vi "Insert Panel at Index.vi"(8 "error in (no error)":errorcluster, 9 "2D Index":T1, 10 "ArrayPanel":refnum<class "ArrayPanel.lvclass">, 11 "2DArrayManager in":refnum<class "2DArrayManager.lvclass">) -> (0 "error out":errorcluster, 1 "Element Replaced":bool, 2 "Replaced Element":refnum<class "ArrayPanel.lvclass">, 3 "2DArrayManager out":refnum<class "2DArrayManager.lvclass">)   [LabVIEW 2020, in "OOPanel.lvlib" / "2DArrayManager.lvclass"]
uses:
  2DArrayManager.lvclass
  ArrayPanel/ArrayPanel.lvclass
  2D Index.ctl
  2DArrayManager.lvclass/2DArrayManager.ctl
  ArrayPanel/ArrayPanel.lvclass/ArrayPanel.ctl
  ec524e60-b0c9-4dc9-b7a4-63c787fc97ef.vi
  <vilib>/Comparison/Equal/Equal Functor/Equal Functor.lvclass
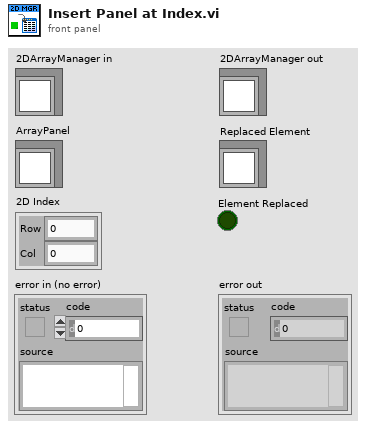
[diagram p1: front panel]
types:
  T1 = typedef "OOPanel.lvlib/2DArrayManager.lvclass/2D Index.ctl" = cluster{"Row":i32, "Col":i32}
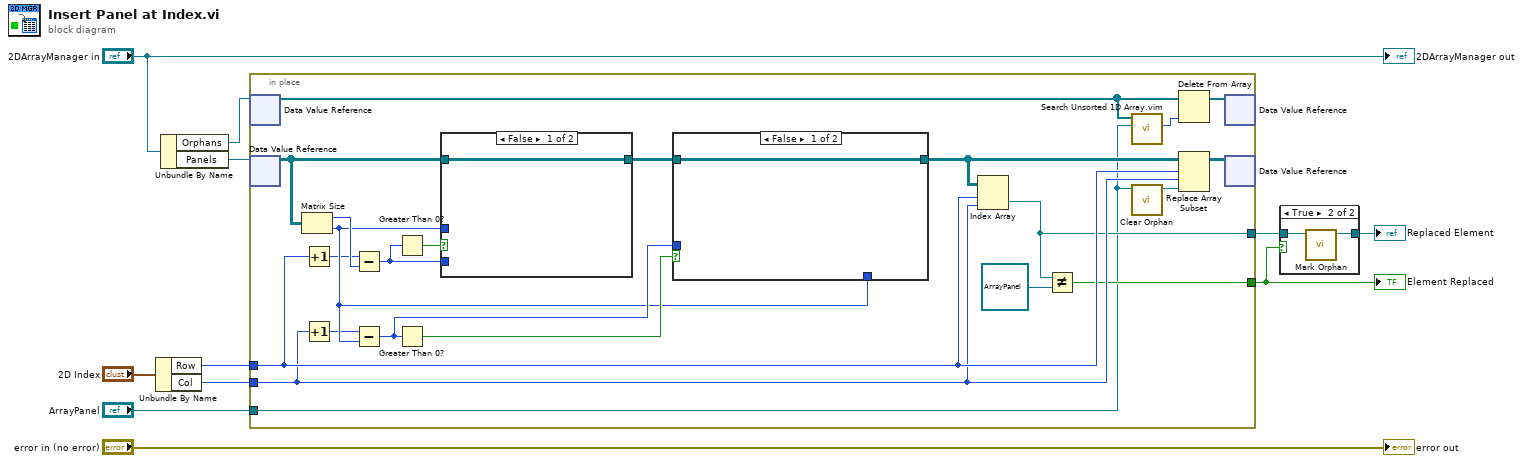
[diagram p0: block diagram]
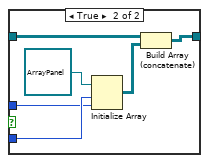
[diagram p2: hidden frame]
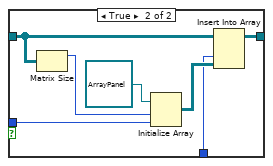
[diagram p3: hidden frame]
diagram:
  n1 = Unbundle By Name("2D Index") -> ("Row"=w7:i32, "Col"=w6:i32)
  n2 = Unbundle By Name("2DArrayManager in") -> ("Orphans"=w1:refnum<data-value>, "Panels"=w9:refnum<data-value>)
  n3 = in-place {
    in-place-border: w7 -> [w23]
    in-place-border: w6 -> [w22]
    in-place-border: "ArrayPanel" -> [w17]
    in-place-border: [w20] -> w4
    in-place-border: [w19] -> w3
    n4 = in-place-dvr #1(w1) -> (w16:refnum<class "ArrayPanel.lvclass">[])  [unwired: 1 out]
    n5 = in-place-dvr #2(w9) -> (w30:refnum<class "ArrayPanel.lvclass">[][])  [unwired: 1 out]
    n6 = Matrix Size(0:w30) -> (1:w33:i32, 2:w25:i32)
    n7 = Increment(x=w23) -> (x+1=w13:i32)
    n8 = Increment(x=w22) -> (x+1=w12:i32)
    n9 = Subtract(x=w13, y=w33) -> (x-y=w31:i32)
    n10 = Subtract(x=w12, y=w25) -> (x-y=w26:i32)
    n11 = Greater Than 0?(x=w31) -> (x > 0?=w32:bool)
    n12 = Greater Than 0?(x=w26) -> (x > 0?=w27:bool)
    n13 = case shown="False" w32 {
      tunnel: w31 -> [_ w40]
      tunnel: w30 -> [w34 w37]
      tunnel: w25 -> [_ w39]
      tunnel: [w34 w35] -> w29
      frame False {
      }
      frame True {
        n14 = Initialize Array(refnum<class "ArrayPanel.lvclass"> refnum ("OOPanel.lvlib:ArrayPanel.lvclass"), w40, w39) -> (w36:refnum<class "ArrayPanel.lvclass">[][])
        n15 = Build Array (concatenate)(w37, w36) -> (w35:refnum<class "ArrayPanel.lvclass">[][])
      }
    }
    n16 = case shown="False" w27 {
      tunnel: w29 -> [w41 w45]
      tunnel: [w41 w43] -> w24
      tunnel: w26 -> [_ w46]
      tunnel: w25 -> [_ w42]
      frame False {
      }
      frame True {
        n17 = Matrix Size(0:w45) -> (1:w47:i32)  [unwired: 1 out]
        n18 = Initialize Array(refnum<class "ArrayPanel.lvclass"> refnum ("OOPanel.lvlib:ArrayPanel.lvclass"), w47, w46) -> (w44:refnum<class "ArrayPanel.lvclass">[][])
        n19 = Insert Into Array(array=w45, index (col)=w42, new element=w44) -> (w43:refnum<class "ArrayPanel.lvclass">[][])  [unwired: 1 in]
      }
    }
    n20 = Index Array(array=w24, index (row)=w23, index (col)=w22) -> (element=w19:refnum<class "ArrayPanel.lvclass">)
    n21 = Not Equal?(x=w19, y=refnum<class "ArrayPanel.lvclass"> refnum ("OOPanel.lvlib:ArrayPanel.lvclass")) -> (x != y?=w20:bool)
    n22 = call "Search Unsorted 1D Array.vim"("element"=w17, "unsorted 1D array"=w16) -> ("index of element"=w15:i32)  [unwired: 9 in]
    n23 = call "Clear Orphan.vi"("ArrayPanel in"=w17) -> ("ArrayPanel out"=w18:refnum<class "ArrayPanel.lvclass">)  [unwired: 9 in, 1 out]
    n24 = Delete From Array(array=w16, index=w15) -> (array with subset deleted=w14:refnum<class "ArrayPanel.lvclass">[])  [unwired: 1 in, 1 out]
    n25 = Replace Array Subset(array=w24, new element=w18, index (row)=w23, index (col)=w22) -> (w28:refnum<class "ArrayPanel.lvclass">[][])
    n26 = in-place-dvr #1(w14) -> ()  [unwired: 2 out]
    n27 = in-place-dvr #2(w28) -> ()  [unwired: 2 out]
  }
  "Element Replaced" <- w4
  n28 = case shown="True" w4 {
    tunnel: w3 -> [_ w50]
    tunnel: [_ w49] -> w2
    frame False {
    }
    frame True {
      n29 = call "Mark Orphan.vi"("ArrayPanel in"=w50) -> ("ArrayPanel out"=w49:refnum<class "ArrayPanel.lvclass">)  [unwired: 9 in, 1 out]
    }
  }
  "Replaced Element" <- w2
  "error out" <- "error in (no error)"
  "2DArrayManager out" <- "2DArrayManager in"
